vi "Adjust Splitter.vi"(8 "error in":errorcluster, 9 "Show":bool, 10 "Splitter Info":T1, 11 "Engine in":refnum<class "Engine.lvclass">) -> (0 "error out":errorcluster, 3 "Engine out":refnum<class "Engine.lvclass">)   [LabVIEW 2023, in "Engine.lvlib" / "Engine.lvclass"]
doc: "This override VI allows ancestor classes to appropriately move splitter positions so the UI fits within the designated pane."
uses:
  Project/Engine.lvclass
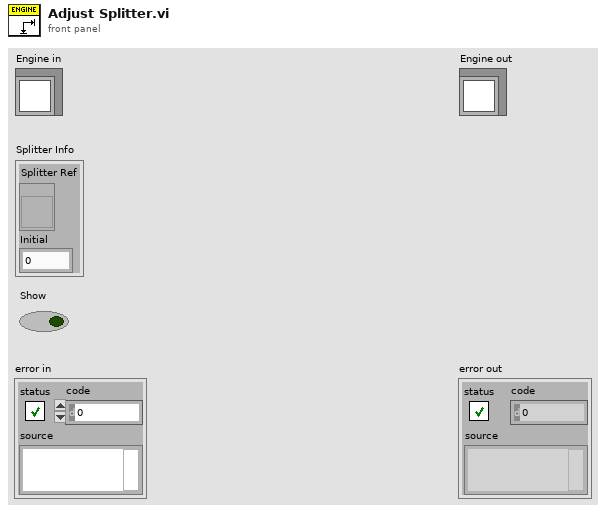
[diagram p1: front panel]
types:
  T1 = cluster{"Splitter Ref":refnum<vi>, "Initial":i32}
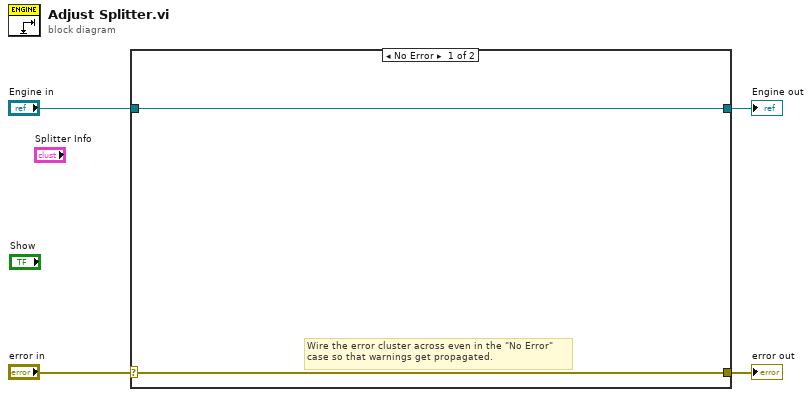
[diagram p0: block diagram]
diagram:
  n1 = case shown="No Error" "error in" {
    selector: "error in" -> [w5 w8]
    tunnel: [w5 w8] -> w3
    tunnel: [w6 w7] -> w1
    tunnel: "Engine in" -> [w6 w7]
    frame No Error {
      # "Wire the error cluster across even in the \"No Error\"\ncase so that warnings get propagated."
    }
    frame Error {
    }
  }
  "error out" <- w3
  "Engine out" <- w1
